vi "Pump Status.vi"(8 "error in (no error)":errorcluster, 11 "State in":T1={"State"=enum."Idle", "Start Time"=timestamp(0 s since 1904-01-01), "Configuration"={"Cycle Period"=0.0, "Ismatech"={"VISA resource name"="", "Simulated?"=FALSE, "Pump Number"=1.0, "Reverse?"=FALSE}, "Masterflex"={"VISA resource name"="", "Simulated?"=FALSE, "Pump Number"=1.0, "Reverse?"=FALSE}, "Mettler"={"VISA resource name"="", "Simulated?"=FALSE}, "Bronkhorst M13 Flow Meter"={"VISA resource name"="", "Simulated?"=FALSE}, "PID 2 Parameters"={"Input Device"=enum."Bronkhorst M13", "Output Device"=enum."Ismatec ISM 831C", "Setpoint"=0.0, "PID gains"={"proportional gain (Kc)"=1.0, "integral time (Ti, min)"=0.01, "derivative time (Td, min)"=0.0}}, "Manual Entry"=0.0, "Auto?"=TRUE, "output range"={"output high"=100.0, "output low"=0.0}, "Bronkhorst M14"={"VISA resource name"="", "Simulated?"=FALSE}, "Tacmina Settings"={"Analog DAQ Task"="", "Digital DAQ Task"=""}, "KNF SIMDOS Settings"={"VISA resource name"="", "Simulated?"=TRUE}, "ASIA Pump C"={"ASIA Pump #"=0, "channel"=0, "Simulated"=FALSE}, "VICI Settings"={"VISA resource name"="", "Simulated?"=FALSE, "Pump Letter"="", "Reverse?"=FALSE}, "FLOM Settings"={"VISA resource name"="", "Simulated?"=TRUE, "Pump Number"=0.0}, "SSI PR Settings"={"VISA resource name"="", "Simulated?"=FALSE}}, "Current Time"=timestamp(0 s since 1904-01-01), "PID 1 Parameters"={"Setpoint"=0.0, "PID gains"={"proportional gain (Kc)"=1.0, "integral time (Ti, min)"=0.01, "derivative time (Td, min)"=0.0}}, "First Iteration"=FALSE, "Data"={"Flowmeter Output"=0.0, "Density"=0.0, "FL Temp"=0.0, "Scale Output (g)"=0.0, "Scale Rate of Change (g/min)"=0.0, "PID 1 Output"=0.0, "PID 2 Process Variable"=0.0, "PID 2 output"=0.0, "Pump Flow"=0.0, "Pump Pressure"=0.0}, "Process Name"="", "Pump On?"=enum."Off", "Input Error"=FALSE, "Output Error"=FALSE, "Log Started"=FALSE, "Current Setpoint"=0.0} {"PID 1 Parameters"."PID gains"."derivative time (Td, min)" format="%.3f"; "PID 1 Parameters"."PID gains"."integral time (Ti, min)" format="%.3f"; "PID 1 Parameters"."PID gains"."proportional gain (Kc)" format="%.3f"; "Configuration"."output range"."output low" min=0.0 max=100.0 format="%.2f"; "Configuration"."output range"."output high" format="%.2f"; "Configuration"."PID 2 Parameters"."PID gains"."derivative time (Td, min)" format="%.3f"; "Configuration"."PID 2 Parameters"."PID gains"."integral time (Ti, min)" format="%.3f"; "Configuration"."PID 2 Parameters"."PID gains"."proportional gain (Kc)" format="%.3f"; "Configuration"."ASIA Pump C"."channel" min=0 max=1 step=1; "Configuration"."Ismatech"."Pump Number" min=1.0 max=20.0 step=1.0; "Configuration"."Masterflex"."Pump Number" min=1.0 max=20.0 step=1.0}) -> (0 "error out":errorcluster, 3 "State out":T1={"State"=enum."Idle", "Start Time"=timestamp(0 s since 1904-01-01), "Configuration"={"Cycle Period"=0.0, "Ismatech"={"VISA resource name"="", "Simulated?"=FALSE, "Pump Number"=1.0, "Reverse?"=FALSE}, "Masterflex"={"VISA resource name"="", "Simulated?"=FALSE, "Pump Number"=1.0, "Reverse?"=FALSE}, "Mettler"={"VISA resource name"="", "Simulated?"=FALSE}, "Bronkhorst M13 Flow Meter"={"VISA resource name"="", "Simulated?"=FALSE}, "PID 2 Parameters"={"Input Device"=enum."Bronkhorst M13", "Output Device"=enum."Ismatec ISM 831C", "Setpoint"=0.0, "PID gains"={"proportional gain (Kc)"=1.0, "integral time (Ti, min)"=0.01, "derivative time (Td, min)"=0.0}}, "Manual Entry"=0.0, "Auto?"=TRUE, "output range"={"output high"=100.0, "output low"=0.0}, "Bronkhorst M14"={"VISA resource name"="", "Simulated?"=FALSE}, "Tacmina Settings"={"Analog DAQ Task"="", "Digital DAQ Task"=""}, "KNF SIMDOS Settings"={"VISA resource name"="", "Simulated?"=TRUE}, "ASIA Pump C"={"ASIA Pump #"=0, "channel"=0, "Simulated"=FALSE}, "VICI Settings"={"VISA resource name"="", "Simulated?"=FALSE, "Pump Letter"="", "Reverse?"=FALSE}, "FLOM Settings"={"VISA resource name"="", "Simulated?"=TRUE, "Pump Number"=0.0}, "SSI PR Settings"={"VISA resource name"="", "Simulated?"=FALSE}}, "Current Time"=timestamp(0 s since 1904-01-01), "PID 1 Parameters"={"Setpoint"=0.0, "PID gains"={"proportional gain (Kc)"=1.0, "integral time (Ti, min)"=0.01, "derivative time (Td, min)"=0.0}}, "First Iteration"=FALSE, "Data"={"Flowmeter Output"=0.0, "Density"=0.0, "FL Temp"=0.0, "Scale Output (g)"=0.0, "Scale Rate of Change (g/min)"=0.0, "PID 1 Output"=0.0, "PID 2 Process Variable"=0.0, "PID 2 output"=0.0, "Pump Flow"=0.0, "Pump Pressure"=0.0}, "Process Name"="", "Pump On?"=enum."Off", "Input Error"=FALSE, "Output Error"=FALSE, "Log Started"=FALSE, "Current Setpoint"=0.0} {"PID 1 Parameters"."PID gains"."derivative time (Td, min)" format="%.3f"; "PID 1 Parameters"."PID gains"."integral time (Ti, min)" format="%.3f"; "PID 1 Parameters"."PID gains"."proportional gain (Kc)" format="%.3f"; "Configuration"."output range"."output low" min=0.0 max=100.0 format="%.2f"; "Configuration"."output range"."output high" format="%.2f"; "Configuration"."PID 2 Parameters"."PID gains"."derivative time (Td, min)" format="%.3f"; "Configuration"."PID 2 Parameters"."PID gains"."integral time (Ti, min)" format="%.3f"; "Configuration"."PID 2 Parameters"."PID gains"."proportional gain (Kc)" format="%.3f"; "Configuration"."ASIA Pump C"."channel" min=0 max=1 step=1; "Configuration"."Ismatech"."Pump Number" min=1.0 max=20.0 step=1.0; "Configuration"."Masterflex"."Pump Number" min=1.0 max=20.0 step=1.0})   [LabVIEW 2018]
uses:
  Measure Instrument/State Cluster.ctl
  Measure Instrument/State Enum.ctl
  Feed Module/Controls/Feed Module Settings Cluster.ctl
  Ismatec ISM 831C/Controls/Ismatech Settings Cluster.ctl
  Masterflex 7550-30/Controls/Settings Cluster.ctl
  Mettler Toledo/Controls/Settings Cluster.ctl
  Bronkhorst M13 Flow Meter/Settings Cluster.ctl
  Measure Instrument/PID 2 Parameters Cluster.ctl
  Measure Instrument/PID Input Enum.ctl
  Measure Instrument/PID 2 Output Enum.ctl
  Tacmina QI/Tacmina QI DAQ Setting.ctl
  KNF Pump/Settings Cluster plus SIMDOS.ctl
  ASIA Pump/Pump Settings.ctl
  VICI M50 Party Mode/Settings Cluster.ctl
  FLOM Pump/Settings Cluster.ctl
  SSI PR Class/SSI PR Settings Cluster.ctl
  Measure Instrument/PID 1 Parameters Cluster.ctl
  Tag VIs/Tag FGV Operation Enum.ctl
  Ismatec ISM 831C/Ismatec ISM 831C.lvlib
  Masterflex 7550-30/Masterflex 7550-30.lvlib
  Measure Instrument/Feed Module Engine.lvlib
  Shared Variables/Dynamic Shared Variables.lvlib
  Tacmina QI/Tacmina QI.lvlib
  KNF Pump/KNF SIMDOS.lvlib
  ASIA Pump.lvlib
  VICI M50 Party Mode/VICI M6 M50 Party Mode.lvlib
  FLOM Pump/FLOM Pump.lvlib
  SSI PR Class/SSI PR Pump.lvlib
  Mettler Toledo/Mettler Toledo.lvlib
  Bronkhorst M13 Flow Meter/Bronkhorst M13 Flow Meter.lvlib
  Feed Module/Feed Module.lvlib
panel:
  # "Output Instruments"
  # "Input Instruments"
  # "Output Instruments"
  # "Input Instruments"
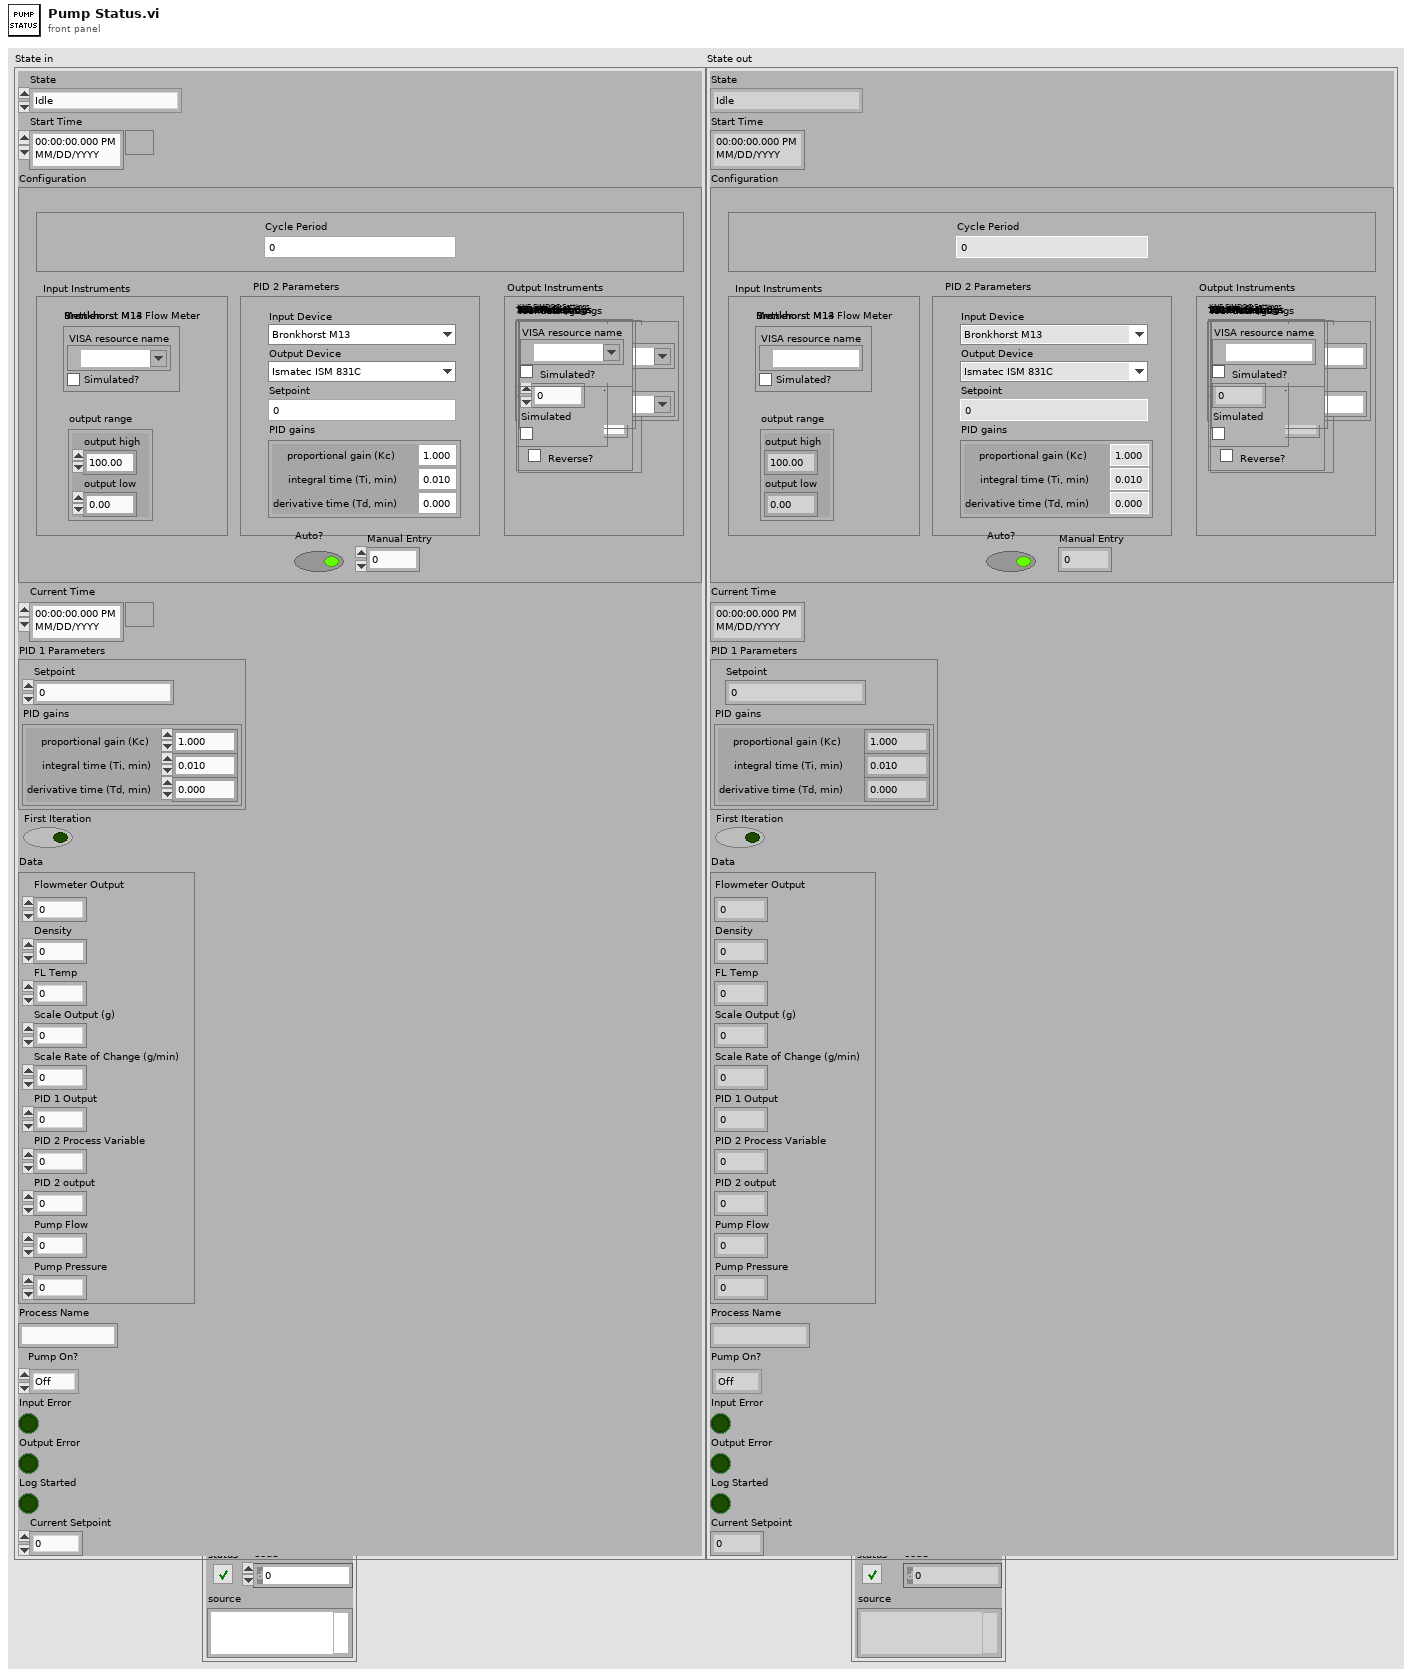
[diagram p1: front panel]
types:
  T1 = typedef "Feed Module.lvlib/Feed Module Engine.lvlib/State Cluster.ctl" = cluster{"State":T2, "Start Time":timestamp, "Configuration":T3, "Current Time":timestamp, "PID 1 Parameters":T17, "First Iteration":bool, "Data":cluster{"Flowmeter Output":dbl, "Density":dbl, "FL Temp":dbl, "Scale Output (g)":dbl, "Scale Rate of Change (g/min)":dbl, "PID 1 Output":dbl, "PID 2 Process Variable":dbl, "PID 2 output":dbl, "Pump Flow":dbl, "Pump Pressure":dbl}, "Process Name":string, "Pump On?":enum16{"Off", "On", "Not Initialized"}, "Input Error":bool, "Output Error":bool, "Log Started":bool, "Current Setpoint":dbl}
  T2 = typedef "Feed Module.lvlib/Feed Module Engine.lvlib/State Enum.ctl" = enum16{"Measuring", "Idle", "Paused"}
  T3 = typedef "Feed Module.lvlib/Feed Module Settings Cluster.ctl" = cluster{"Cycle Period":dbl, "Ismatech":T4, "Masterflex":T5, "Mettler":T6, "Bronkhorst M13 Flow Meter":T7, "PID 2 Parameters":T8, "Manual Entry":dbl, "Auto?":bool, "output range":cluster{"output high":dbl, "output low":dbl}, "Bronkhorst M14":T6, "Tacmina Settings":T11, "KNF SIMDOS Settings":T12, "ASIA Pump C":T13, "VICI Settings":T14, "FLOM Settings":T15, "SSI PR Settings":T16}
  T4 = typedef "Ismatec ISM 831C.lvlib/Ismatech Settings Cluster.ctl" = cluster{"VISA resource name":refnum<visa-resource-name>, "Simulated?":bool, "Pump Number":dbl, "Reverse?":bool}
  T5 = typedef "Masterflex 7550-30.lvlib/Settings Cluster.ctl" = cluster{"VISA resource name":refnum<visa-resource-name>, "Simulated?":bool, "Pump Number":dbl, "Reverse?":bool}
  T6 = typedef "Mettler Toledo.lvlib/Settings Cluster.ctl" = cluster{"VISA resource name":refnum<visa-resource-name>, "Simulated?":bool}
  T7 = typedef "Bronkhorst M13 Flow Meter.lvlib/Settings Cluster.ctl" = cluster{"VISA resource name":refnum<visa-resource-name>, "Simulated?":bool}
  T8 = typedef "PID 2 Parameters Cluster.ctl" = cluster{"Input Device":T9, "Output Device":T10, "Setpoint":dbl, "PID gains":cluster{"proportional gain (Kc)":dbl, "integral time (Ti, min)":dbl, "derivative time (Td, min)":dbl}}
  T9 = typedef "PID Input Enum.ctl" = enum16{"Default", "Bronkhorst M13", "Bronkhorst M14", "Scale Rate of Change"}
  T10 = typedef "PID 2 Output Enum.ctl" = enum16{"Default", "Ismatec ISM 831C", "Masterflex 7550-30", "VICI", "Tacmina QI", "KNF SIMDOS", "ASIA Type C", "FLOM UI-22-11", "SSI PR"}
  T11 = typedef "Tacmina QI.lvlib/Tacmina QI DAQ Setting.ctl" = cluster{"Analog DAQ Task":refnum<k21>, "Digital DAQ Task":refnum<k21>}
  T12 = typedef "KNF SIMDOS.lvlib/Settings Cluster plus SIMDOS.ctl" = cluster{"VISA resource name":refnum<visa-resource-name>, "Simulated?":bool}
  T13 = typedef "ASIA Pump.lvlib/Pump Settings.ctl" = cluster{"ASIA Pump #":i32, "channel":i32, "Simulated":bool}
  T14 = typedef "VICI M6 M50 Party Mode.lvlib/Settings Cluster.ctl" = cluster{"VISA resource name":refnum<visa-resource-name>, "Simulated?":bool, "Pump Letter":string, "Reverse?":bool}
  T15 = typedef "FLOM Pump.lvlib/Settings Cluster.ctl" = cluster{"VISA resource name":refnum<visa-resource-name>, "Simulated?":bool, "Pump Number":dbl}
  T16 = typedef "SSI PR Pump.lvlib/SSI PR Settings Cluster.ctl" = cluster{"VISA resource name":refnum<visa-resource-name>, "Simulated?":bool}
  T17 = typedef "PID 1 Parameters Cluster.ctl" = cluster{"Setpoint":dbl, "PID gains":cluster{"proportional gain (Kc)":dbl, "integral time (Ti, min)":dbl, "derivative time (Td, min)":dbl}}
  T18 = typedef "Tag FGV Operation Enum.ctl" = enum16{"Init", "Set Notification Queue", "Create Tag", "Commit", "Write Tag (Numeric)", "Write Tag (Boolean)", "Read All Tags", "Read One Tag", "Delete Tag Category", "Set Alarm Parameters (Numeric)", "Set Alarm Parameters (Boolean)", "Enable All Alarms", "Disable All Alarms", "Delete All Tags", "Read Alarms", "Ack Alarm"}
  T19 = typedef "Feed Module.lvlib/Feed Module Tag Names Cluster.ctl" = cluster{"Pump Flow Tag":string, "PID 2 Out Tag":string, "Scale Tag":string, "Density Tag":string, "FL Temp":string, "Input Device Tag":string, "Output Device Tag":string, "Pump's Flow":string, "Pump's Pressure":string, "Overpressure Tag":string}
  T20 = cluster{"alarm URL":string, "set time":timestamp, "set user":string, "ack time":timestamp, "ack user":string, "clear time":timestamp, "clear user":string, "setpoint":dbl, "value":dbl, "priority":u32, "alarm area":string, "alarm description":string, "ack comment":string, "event?":bool, "Refnum":u64}[]
  T21 = typedef "Dynamic Shared Variables.lvlib/Alarm Cluster (UI).ctl" = cluster{"Color Box":u32, "Name":string, "Ack":bool}
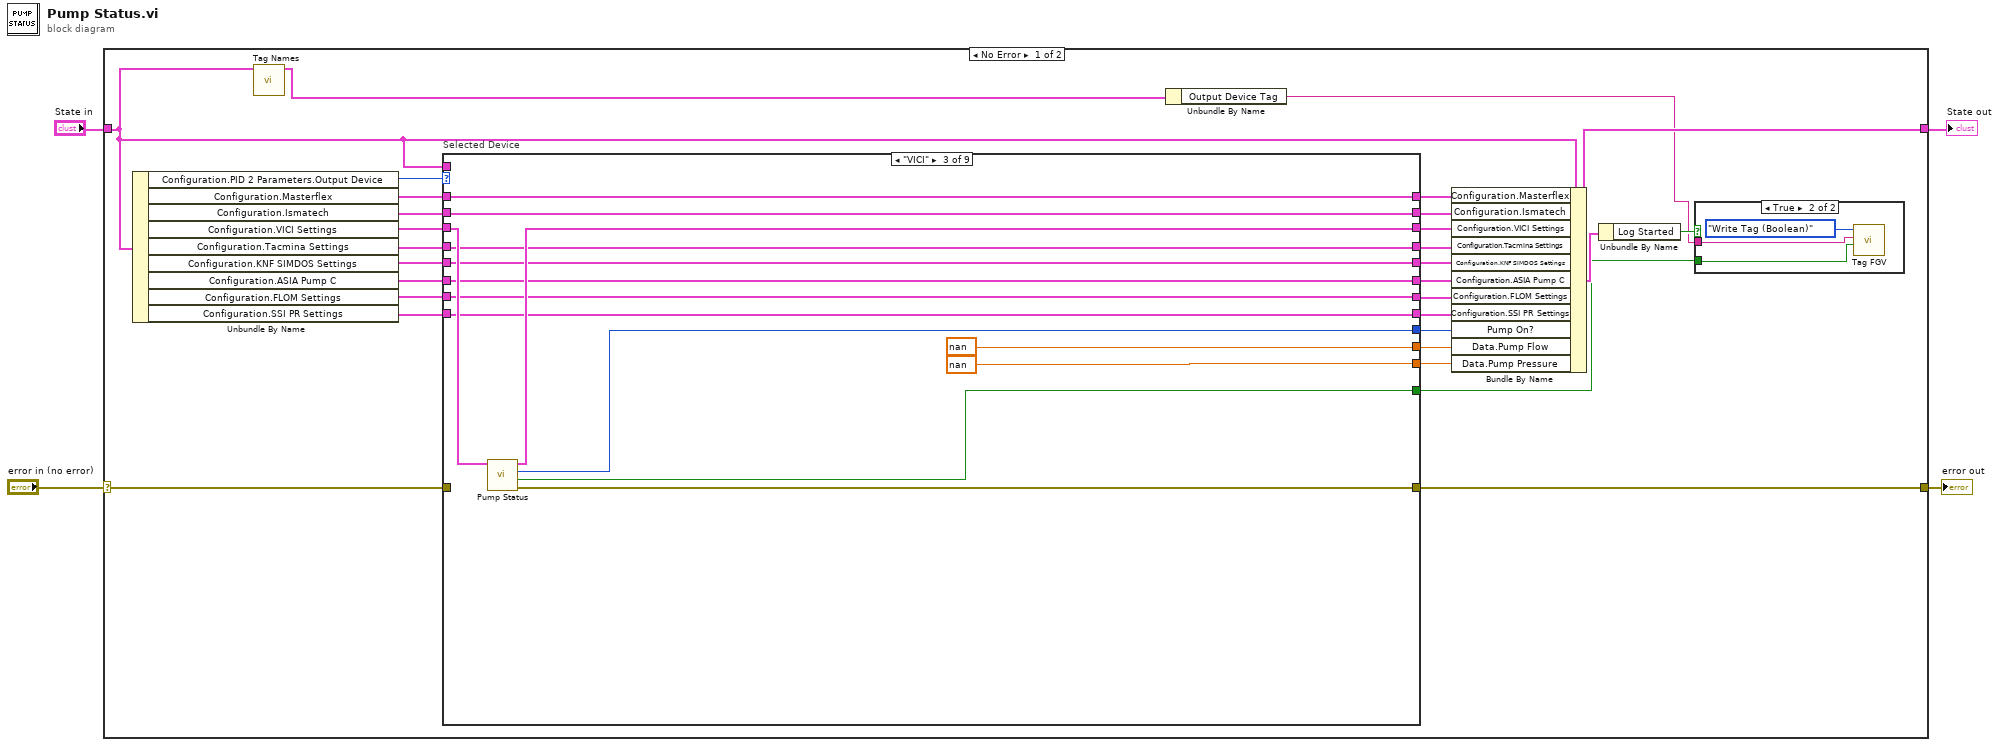
[diagram p0: block diagram]
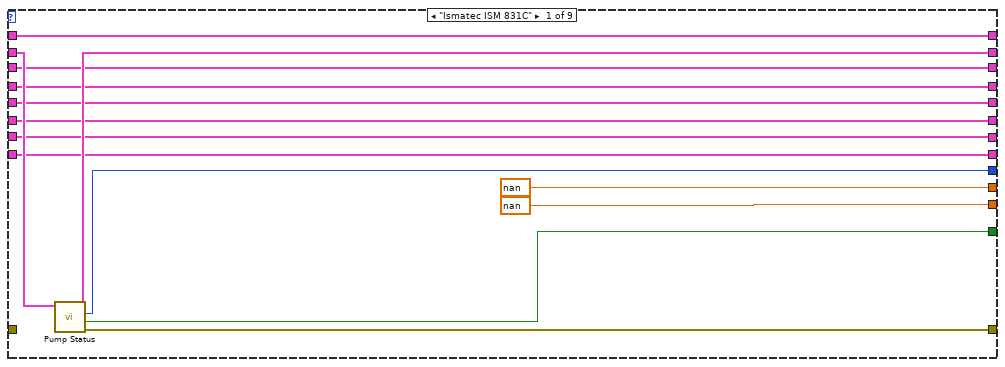
[diagram p2: hidden frame]
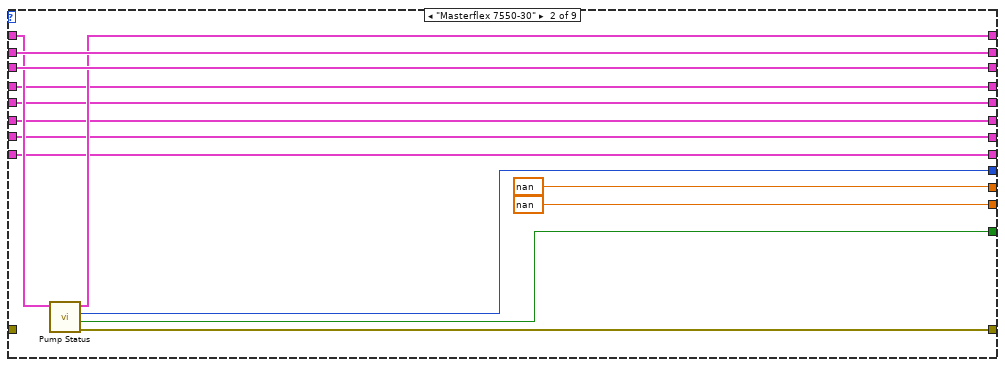
[diagram p3: hidden frame]
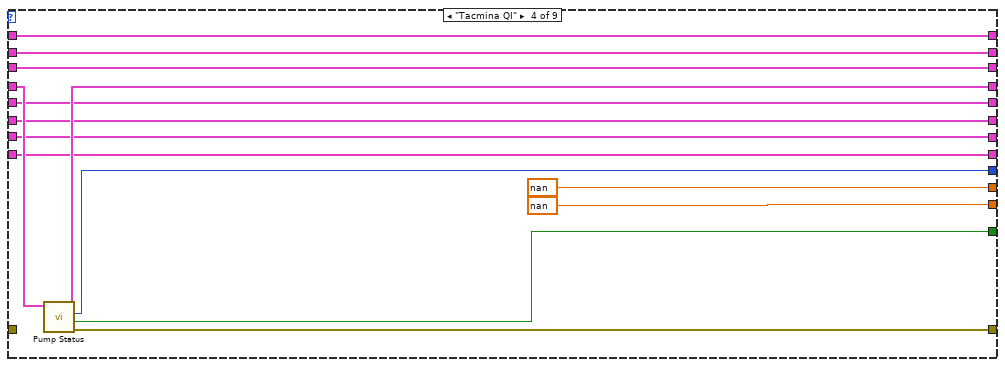
[diagram p4: hidden frame]
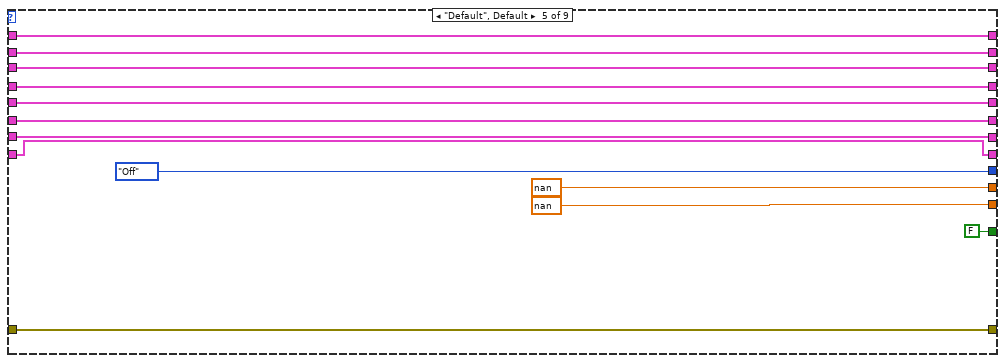
[diagram p5: hidden frame]
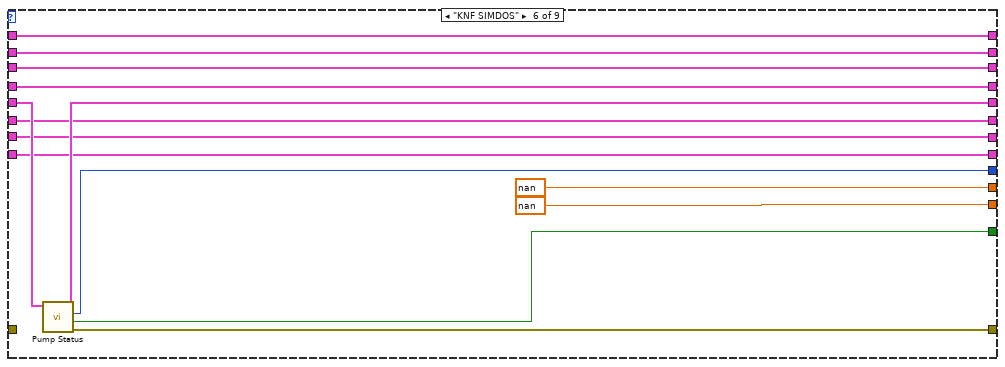
[diagram p6: hidden frame]
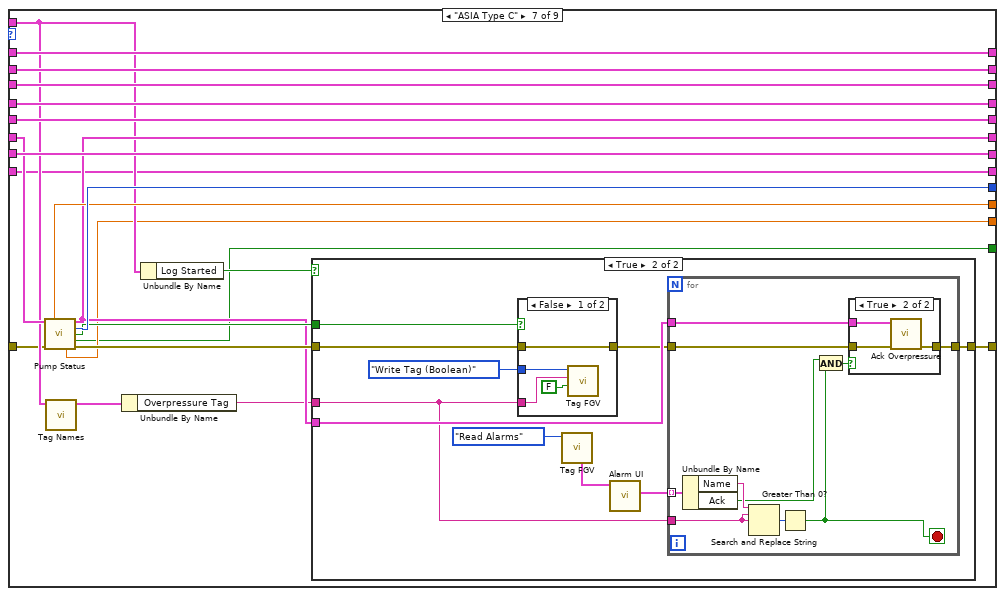
[diagram p7: hidden frame]
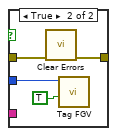
[diagram p10: hidden frame]
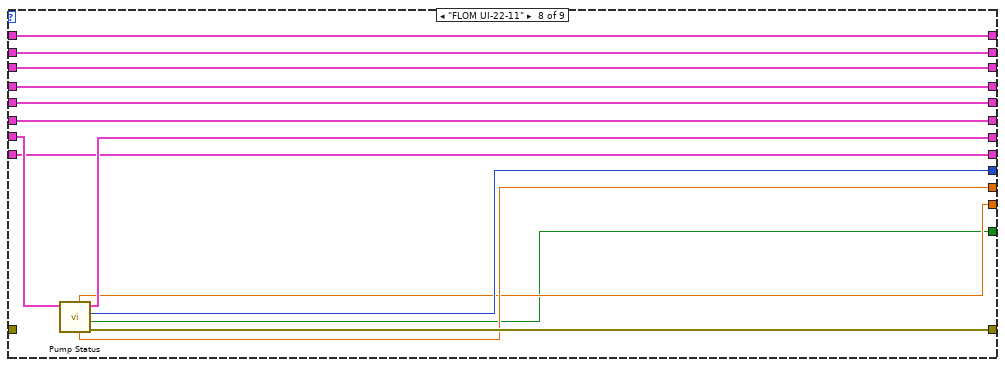
[diagram p11: hidden frame]
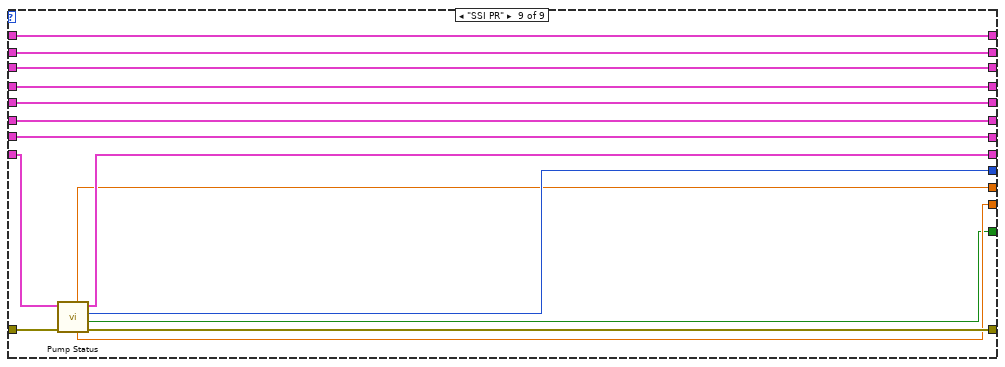
[diagram p12: hidden frame]
diagram:
  n1 = case shown="No Error" "error in (no error)" {
    selector: "error in (no error)" -> [w21 w203]
    tunnel: [w25 w203] -> w3
    tunnel: "State in" -> [w26 w202]
    tunnel: [w32 w202] -> w1
    frame No Error {
      n2 = Unbundle By Name(w26) -> ("Configuration.PID 2 Parameters.Output Device"=w10:T10, "Configuration.Masterflex"=w30:T5, "Configuration.Ismatech"=w29:T4, "Configuration.VICI Settings"=w28:T14, "Configuration.Tacmina Settings"=w24:T11, "Configuration.KNF SIMDOS Settings"=w23:T12, "Configuration.ASIA Pump C"=w22:T13, "Configuration.FLOM Settings"=w27:T15, "Configuration.SSI PR Settings"=w7:T16)
      n3 = call "Tag Names.vi"("State in"=w26) -> ("Feed Module Tag Names"=w9:T19)  [unwired: 6 in, 4 out]
      n4 = case "Selected Device" shown="\"VICI\"" w10 {
        tunnel: w30 -> [w46 w56 w73 w88 w101 w115 w136 w183 w188]
        tunnel: [w46 w57 w73 w88 w101 w115 w136 w183 w188] -> w20
        tunnel: w29 -> [w44 w60 w74 w87 w100 w114 w135 w182 w198]
        tunnel: [w45 w58 w70 w84 w91 w111 w124 w177 w190] -> w25
        tunnel: w21 -> [_ _ _ _ w91 _ w121 _ w191]
        tunnel: [w43 w60 w74 w87 w100 w114 w135 w182 w198] -> w19
        tunnel: w28 -> [w41 w59 w71 w86 w99 w113 w134 w181 w197]
        tunnel: [w41 w59 w72 w86 w99 w113 w134 w181 w197] -> w18
        tunnel: w24 -> [w42 w55 w69 w85 w98 w112 w133 w180 w196]
        tunnel: [w42 w55 w69 w83 w98 w112 w133 w180 w196] -> w17
        tunnel: [w40 w54 w68 w82 w97 w110 w132 w179 w195] -> w16
        tunnel: w23 -> [w40 w54 w68 w82 w97 w109 w132 w179 w195]
        tunnel: [w39 w52 w67 w81 enum16{"Off", "On", "Not Initialized"}."Off" ("Pump On?") w108 w129 w174 w187] -> w6
        tunnel: [w38 w53 w66 w80 w95 w107 w123 w178 w194] -> w15
        tunnel: w22 -> [w38 w53 w66 w80 w95 w107 w130 w178 w194]
        tunnel: [w37 w51 w65 w79 w94 w106 w131 w176 w193] -> w14
        tunnel: w27 -> [w37 w51 w65 w79 w94 w106 w131 w175 w193]
        tunnel: [nan ("Pressure") nan ("Pressure") nan ("Pressure") nan ("Pressure") nan ("Pressure") nan ("Pressure") w127 w173 w186] -> w13
        tunnel: w26 -> [_ _ _ _ _ _ w122 _ _]
        tunnel: [nan ("Flow Rate") nan ("Flow Rate") nan ("Flow Rate") nan ("Flow Rate") nan ("Flow Rate") nan ("Flow Rate") w120 w172 w185] -> w12
        tunnel: [w34 w48 w62 w76 FALSE ("Connection Error") w103 w119 w171 w184] -> w11
        tunnel: w7 -> [w33 w47 w61 w75 w89 w102 w116 w170 w192]
        tunnel: [w33 w47 w61 w75 w89 w102 w116 w170 w189] -> w5
        frame "Ismatec ISM 831C" {
          n5 = call "Pump Status.vi"("Ismatech Settings"=w44) -> ("error out"=w45:errorcluster, "Connection Error"=w34:bool, "Pump On?"=w39:enum16{"Off", "On", "Not Initialized"}, "Ismatech Settings"=w43:T4)  [unwired: 7 in]
        }
        frame "Masterflex 7550-30" {
          n6 = call "Pump Status.vi"("Masterflex Settings in"=w56) -> ("error out"=w58:errorcluster, "Connection Error"=w48:bool, "Pump On?"=w52:enum16{"Off", "On", "Not Initialized"}, "Masterflex Settings out"=w57:T5)  [unwired: 7 in]
        }
        frame "VICI" {
          n7 = call "Pump Status.vi"("VICI Settings"=w71) -> ("error out"=w70:errorcluster, "Connection Error"=w62:bool, "Pump On?"=w67:enum16{"Off", "On", "Not Initialized"}, "VICI Settings"=w72:T14)  [unwired: 7 in]
        }
        frame "Tacmina QI" {
          n8 = call "Pump Status.vi"("Tacmina Settings in"=w85) -> ("error out"=w84:errorcluster, "Connection Error"=w76:bool, "Pump On?"=w81:enum16{"Off", "On", "Not Initialized"}, "Tacmina Settings out"=w83:T11)  [unwired: 7 in]
        }
        frame "Default", Default {
        }
        frame "KNF SIMDOS" {
          n9 = call "Pump Status.vi"("KNF Settings"=w109) -> ("error out"=w111:errorcluster, "Connection Error"=w103:bool, "Pump On?"=w108:enum16{"Off", "On", "Not Initialized"}, "KNF Settings"=w110:T12)  [unwired: 7 in]
        }
        frame "ASIA Type C" {
          n10 = call "Pump Status.vi"("ASIA Pump C Settings in"=w130, "error in (no error)"=w121) -> ("pressure"=w127:dbl, "ASIA Pump C Settings out"=w123:T13, "Pump On?"=w129:enum16{"Off", "On", "Not Initialized"}, "Overpressure"=w126:bool, "Connection Error"=w119:bool, "pumpRate"=w120:dbl, "error out"=w128:errorcluster)  [unwired: 5 in, 2 out]
          n11 = call "Tag Names.vi"("State in"=w122) -> ("Feed Module Tag Names"=w118:T19)  [unwired: 6 in, 4 out]
          n12 = Unbundle By Name(w118) -> ("Overpressure Tag"=w117:string)
          n13 = Unbundle By Name(w122) -> ("Log Started"=w125:bool)
          n14 = case shown="True" w125 {
            tunnel: w128 -> [w137 w147]
            tunnel: w126 -> [_ w146]
            tunnel: [w137 w140] -> w124
            tunnel: w123 -> [_ w141]
            tunnel: w117 -> [_ w138]
            frame False {
            }
            frame True {
              n15 = case shown="False" w146 {
                tunnel: Tag_FGV_Operation_Enum."Write Tag (Boolean)" ("Operation") -> [w165 w169]
                tunnel: [w164 w167] -> w139
                tunnel: w147 -> [w164 w168]
                tunnel: w138 -> [w162 _]
                frame False {
                  n16 = call "Tag FGV.vi"("Data"=FALSE, "Tag Name"=w162, "Operation"=w165) -> ()  [unwired: 3 in, 6 out]
                }
                frame True {
                  n17 = call <vilib>:"Clear Errors.vi"("error in (no error)"=w168) -> ("error out"=w167:errorcluster)  [unwired: 5 in, 1 out]
                  n18 = call "Tag FGV.vi"("Data"=TRUE, "Operation"=w169) -> ()  [unwired: 4 in, 6 out]
                }
              }
              n19 = call "Tag FGV.vi"("Operation"=Tag_FGV_Operation_Enum."Read Alarms") -> ("alarms"=w143:T20)  [unwired: 5 in, 5 out]
              n20 = call "Alarm UI.vi"("alarms"=w143) -> ("UI Alarms"=w142:T21[])  [unwired: 9 in, 1 out]
              n21 = for {
                tunnel: w142 -> [w157] mode=indexing
                tunnel: w141 -> [w154]
                tunnel: [w153] -> w140
                tunnel: w139 -> [w152]
                tunnel: w138 -> [w148]
                stop <- w150 stop-if-true
                n22 = Unbundle By Name(w157) -> ("Name"=w156:string, "Ack"=w149:bool)
                n23 = Search and Replace String(input string=w156, search string=w148, replace string=w148) -> (number of replacements=w155:i32)  [unwired: 5 in, 3 out]
                n24 = Greater Than 0?(x=w155) -> (x > 0?=w150:bool)
                n25 = And(x=w149, y=w150) -> (x .and. y?=w151:bool)
                n26 = case shown="True" w151 {
                  tunnel: w154 -> [_ w161]
                  tunnel: [w158 w160] -> w153
                  tunnel: w152 -> [w158 w159]
                  frame False {
                  }
                  frame True {
                    n27 = call "Ack Overpressure.vi"("error in (no error)"=w159, "ASIA Pump C Settings in"=w161) -> ("error out"=w160:errorcluster)  [unwired: 9 in]
                  }
                }
              }
            }
          }
        }
        frame "FLOM UI-22-11" {
          n28 = call "Pump Status.vi"("FLOM Settings In"=w175) -> ("error out"=w177:errorcluster, "Connection Error"=w171:bool, "Pump On?"=w174:enum16{"Off", "On", "Not Initialized"}, "FLOM Settings Out"=w176:T15, "Pressure"=w173:dbl, "Flow Rate"=w172:dbl)  [unwired: 5 in]
        }
        frame "SSI PR" {
          n29 = call "Pump Status.vi"("error in (no error)"=w191, "SSI PR Settings"=w192) -> ("error out"=w190:errorcluster, "Connection Error"=w184:bool, "Pump On?"=w187:enum16{"Off", "On", "Not Initialized"}, "SSI PR Settings"=w189:T16, "Pressure"=w185:dbl, "Flow"=w186:dbl)  [unwired: 4 in]
        }
      }
      n30 = Unbundle By Name(w9) -> ("Output Device Tag"=w8:string)
      n31 = Bundle By Name(cluster=w26, "Configuration.Masterflex"=w20, "Configuration.Ismatech"=w19, "Configuration.VICI Settings"=w18, "Configuration.Tacmina Settings"=w17, "Configuration.KNF SIMDOS Settings"=w16, "Configuration.ASIA Pump C"=w15, "Configuration.FLOM Settings"=w14, "Configuration.SSI PR Settings"=w5, "Pump On?"=w6, "Data.Pump Flow"=w13, "Data.Pump Pressure"=w12) -> (w32:T1)
      n32 = Unbundle By Name(w32) -> ("Log Started"=w31:bool)
      n33 = case shown="True" w31 {
        tunnel: w8 -> [_ w199]
        tunnel: w11 -> [_ w200]
        frame False {
        }
        frame True {
          n34 = call "Tag FGV.vi"("Data"=w200, "Tag Name"=w199, "Operation"=Tag_FGV_Operation_Enum."Write Tag (Boolean)") -> ()  [unwired: 3 in, 6 out]
        }
      }
    }
    frame Error {
    }
  }
  "error out" <- w3
  "State out" <- w1
